vi "dual_color_2D_AFM_synched.vi"() -> ()   [LabVIEW 2017]
uses:
  <vilib>/DAQmx/write.llb/DAQmx Write (Analog DBL 1Chan 1Samp).vi
  <vilib>/DAQmx/write.llb/DAQmx Write (Analog 2D DBL NChan NSamp).vi
  <vilib>/DAQmx/write.llb/DAQmx Write (Analog 1D DBL NChan 1Samp).vi
  <vilib>/DAQmx/create/channels.llb/DAQmx Create Channel (AO-Voltage-Basic).vi
  <vilib>/DAQmx/miscellaneous.llb/DAQmx Fill In Error Info.vi
  <vilib>/DAQmx/configure/timing.llb/DAQmx Timing (Sample Clock).vi
  <vilib>/DAQmx/configure/trigger.llb/DAQmx Start Trigger (Digital Edge).vi
  <resource>/objmgr/daqmx.rc
panel:
  out "Focal Distance (um)":dbl
  out "Diopter":dbl
  in  "ETL3 (v) [4.76V allows light passing through unaltered]":dbl(slide)=4.76 min=-10.0 max=10.0 step=0.01 scale=-10.0..10.0
  in  "Y multiplier":dbl=1.0
  in  "X multiplier":dbl=-1.0
  in  "Y (v)":dbl(slide) min=-10.0 max=10.0 step=0.01 scale=-10.0..10.0
  in  "X (v)":dbl(slide) min=-10.0 max=10.0 step=0.01 scale=-10.0..10.0
  in  "Combined Movement (v)\nEquation: X * X Multiplier + Y * Y Multiplier":dbl(slide) min=-10.0 max=10.0 step=0.01 scale=-10.0..10.0
  out "Expected AFM Frequency (HZ)":dbl
  in  "Listbox 2":i32(listbox)=3
  in  "Listbox":i32(listbox)=1
  in  "Laser 2 (0-10v)":dbl=3.0
  in  "Laser 1 (0-10v)":dbl=3.0
  in  "OFF Time(ms)":dbl=100.0
  in  "ON Time(ms)":dbl=300.0
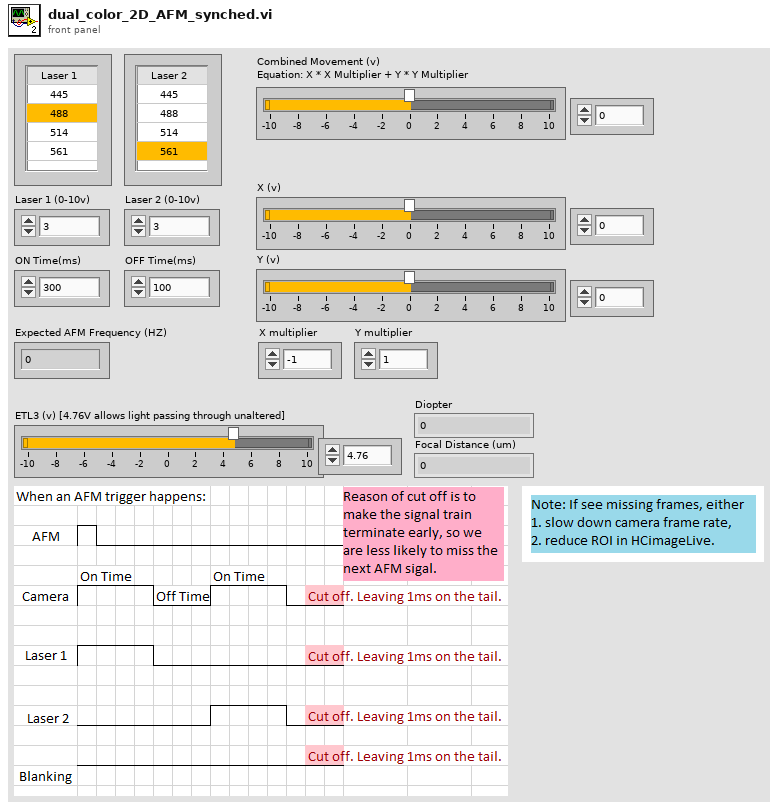
[diagram p1: front panel]
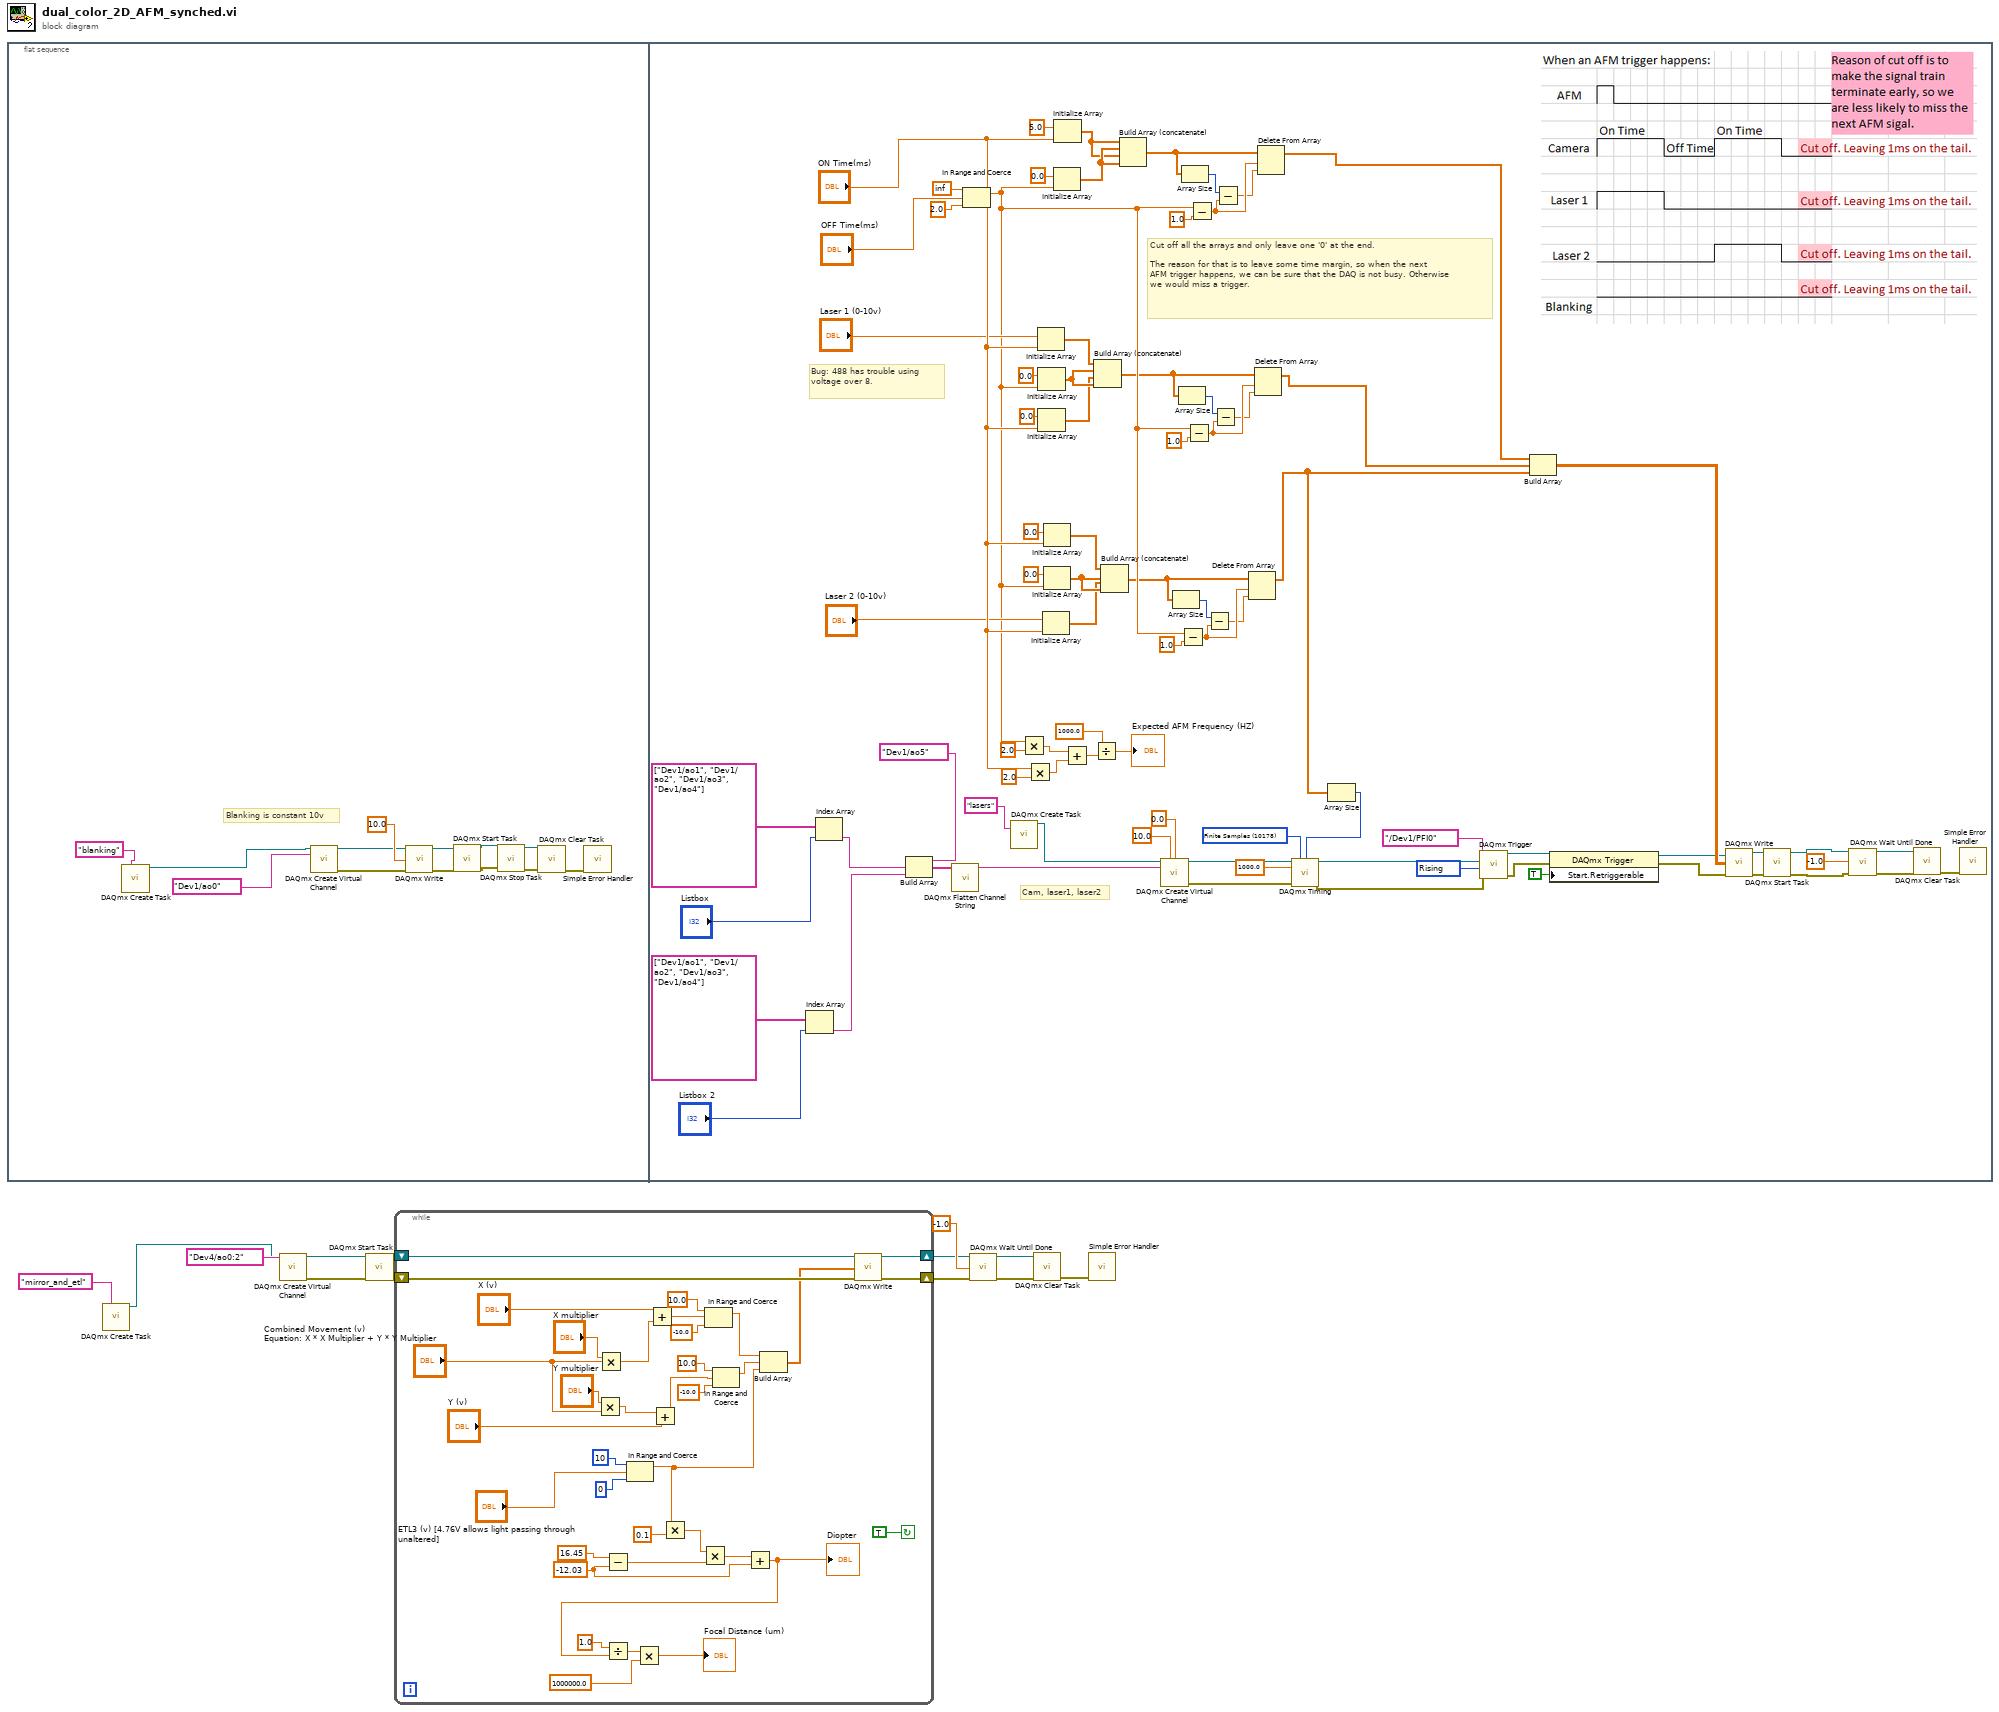
[diagram p0: block diagram]
diagram:
  n1 = flat-sequence {
    frame #0 {
      # "Blanking is constant 10v"
      n2 = call <vilib>:"DAQmx Create Task.vi"("new task name"="blanking" ("name to assign")) -> ("task out"=w16:refnum<k21>)  [unwired: 13 in, 1 out]
      n3 = call-poly <vilib>:"DAQmx Create Virtual Channel.vi"("task in"=w16, "physical channels"=tag "Dev1/ao0") -> ("task out"=w24:refnum<k21>, "error out"=w23:errorcluster)  [unwired: 12 in]
      n4 = call-poly <vilib>:"DAQmx Write.vi"("task/channels in"=w24, "data"=10.0, "error in"=w23) -> ("task out"=w22:refnum<k21>, "error out"=w21:errorcluster)  [unwired: 10 in, 1 out]
      n5 = call <vilib>:"DAQmx Start Task.vi"("task/channels in"=w22, "error in"=w21) -> ("task out"=w15:refnum<k21>, "error out"=w14:errorcluster)  [unwired: 12 in]
      n6 = call <vilib>:"DAQmx Stop Task.vi"("task/channels in"=w15, "error in"=w14) -> ("task out"=w20:refnum<k21>, "error out"=w19:errorcluster)  [unwired: 12 in]
      n7 = call <vilib>:"DAQmx Clear Task.vi"("task in"=w20, "error in"=w19) -> ("error out"=w26:errorcluster)  [unwired: 13 in]
      n8 = call <vilib>:"Simple Error Handler.vi"("error in (no error)"=w26) -> ()  [unwired: 4 in, 5 out]
    }
    frame #1 {
      w43 = 10280 items=["Rising"=10280, "Falling"=10171] ("edge")
      w39 = 10178 items=["Finite Samples"=10178, "Continuous Samples"=10123, "Hardware Timed Single Point"=12522] ("sample mode")
      # "Bug: 488 has trouble using voltage over 8."
      # "Cut off all the arrays and only leave one '0' at the end.\n\nThe reason for that is to leave some time margin, so when the next \nAFM trigger happens, we can be sure that the DAQ is not busy. Otherwise\nwe would miss a trigger."
      # "Cam, laser1, laser2"
      n9 = Index Array(array=tag[] ["Dev1/ao1", "Dev1/ao2", "Dev1/ao3", "Dev1/ao4"], index="Listbox 2") -> (element=w102:tag)
      n10 = Index Array(array=tag[] ["Dev1/ao1", "Dev1/ao2", "Dev1/ao3", "Dev1/ao4"], index="Listbox") -> (element=w101:tag)
      n11 = Build Array(tag "Dev1/ao5" ("physical channels"), w101, w102) -> (w103:tag[])
      n12 = call <vilib>:"DAQmx Flatten Channel String.vi"("names in"=w103) -> ("names out"=w106:string)  [unwired: 13 in, 1 out]
      n13 = In Range and Coerce(upper limit=inf, x="OFF Time(ms)", lower limit=2.0) -> (coerced(x)=w88:dbl)  [unwired: 1 out]
      n14 = call <vilib>:"DAQmx Create Task.vi"("new task name"="lasers" ("name to assign")) -> ("task out"=w108:refnum<k21>)  [unwired: 13 in, 1 out]
      n15 = Multiply(x=w88, y=2.0) -> (x*y=w90:dbl)
      n16 = Multiply(x="ON Time(ms)", y=2.0) -> (x*y=w89:dbl)
      n17 = Initialize Array("Laser 1 (0-10v)", "ON Time(ms)") -> (w59:dbl[])
      n18 = Initialize Array(0.0 ("element"), w88) -> (w61:dbl[])
      n19 = Initialize Array(0.0 ("element"), "ON Time(ms)") -> (w60:dbl[])
      n20 = Initialize Array("Laser 2 (0-10v)", "ON Time(ms)") -> (w67:dbl[])
      n21 = Initialize Array(0.0 ("element"), "ON Time(ms)") -> (w66:dbl[])
      n22 = Initialize Array(0.0 ("element"), w88) -> (w68:dbl[])
      n23 = Initialize Array(0.0 ("element"), w88) -> (w54:dbl[])
      n24 = Initialize Array(5.0 ("element"), "ON Time(ms)") -> (w53:dbl[])
      n25 = Add(x=w90, y=w89) -> (x+y=w91:dbl)
      n26 = Divide(x=1000.0, y=w91) -> (x/y=→"Expected AFM Frequency (HZ)":dbl)
      n27 = Build Array (concatenate)(w59, w61, w60, w61) -> (w65:dbl[])
      n28 = Build Array (concatenate)(w66, w68, w67, w68) -> (w72:dbl[])
      n29 = Build Array (concatenate)(w53, w54, w53, w54) -> (w55:dbl[])
      n30 = call-poly <vilib>:"DAQmx Create Virtual Channel.vi"("task in"=w108, "maximum value"=10.0, "minimum value"=0.0, "physical channels"=w106) -> ("task out"=w80:refnum<k21>, "error out"=w81:errorcluster)  [unwired: 10 in]
      n31 = Array Size(array=w72) -> (size(s)=w69:i32)
      n32 = Array Size(array=w65) -> (size(s)=w62:i32)
      n33 = Subtract(x=w88, y=1.0) -> (x-y=w71:dbl)
      n34 = Array Size(array=w55) -> (size(s)=w56:i32)
      n35 = Subtract(x=w88, y=1.0) -> (x-y=w64:dbl)
      n36 = Subtract(x=w88, y=1.0) -> (x-y=w58:dbl)
      n37 = Subtract(x=w69, y=w71) -> (x-y=w70:dbl)
      n38 = Subtract(x=w62, y=w64) -> (x-y=w63:dbl)
      n39 = Subtract(x=w56, y=w58) -> (x-y=w57:dbl)
      n40 = Delete From Array(array=w72, length=w71, index=w70) -> (array with subset deleted=w95:dbl[])  [unwired: 1 out]
      n41 = Delete From Array(array=w65, length=w64, index=w63) -> (array with subset deleted=w93:dbl[])  [unwired: 1 out]
      n42 = Delete From Array(array=w55, length=w58, index=w57) -> (array with subset deleted=w92:dbl[])  [unwired: 1 out]
      n43 = Array Size(array=w95) -> (size(s)=w107:i32)
      n44 = call-poly <vilib>:"DAQmx Timing.vi"("task/channels in"=w80, "sample mode"=w39, "samples per channel"=w107, "rate"=1000.0, "error in"=w81) -> ("task out"=w82:refnum<k21>, "error out"=w83:errorcluster)  [unwired: 9 in]
      n45 = call-poly <vilib>:"DAQmx Trigger.vi"("task/channels in"=w82, "source"=tag "/Dev1/PFI0", "edge"=w43, "error in"=w83) -> ("task out"=w84:refnum<k21>, "error out"=w87:errorcluster)  [unwired: 10 in]
      n46 = Build Array(w92, w93, w95) -> (w94:dbl[][])
      n47 = property class="DAQmx Trigger"(reference=w84, error in=w87, "Start.Retriggerable"=TRUE) -> (reference out=w85:refnum<k21>, error out=w86:errorcluster)
      n48 = call-poly <vilib>:"DAQmx Write.vi"("task/channels in"=w85, "data"=w94, "error in"=w86) -> ("task out"=w78:refnum<k21>, "error out"=w79:errorcluster)  [unwired: 10 in, 1 out]
      n49 = call <vilib>:"DAQmx Start Task.vi"("task/channels in"=w78, "error in"=w79) -> ("task out"=w77:refnum<k21>, "error out"=w76:errorcluster)  [unwired: 12 in]
      n50 = call <vilib>:"DAQmx Wait Until Done.vi"("task/channels in"=w77, "timeout (sec)"=-1.0, "error in"=w76) -> ("task out"=w74:refnum<k21>, "error out"=w75:errorcluster)  [unwired: 11 in]
      n51 = call <vilib>:"DAQmx Clear Task.vi"("task in"=w74, "error in"=w75) -> ("error out"=w73:errorcluster)  [unwired: 13 in]
      n52 = call <vilib>:"Simple Error Handler.vi"("error in (no error)"=w73) -> ()  [unwired: 4 in, 5 out]
    }
  }
  n53 = call <vilib>:"DAQmx Create Task.vi"("new task name"="mirror_and_etl" ("name to assign")) -> ("task out"=w1:refnum<k21>)  [unwired: 13 in, 1 out]
  n54 = call-poly <vilib>:"DAQmx Create Virtual Channel.vi"("task in"=w1, "physical channels"=tag "Dev4/ao0:2") -> ("task out"=w6:refnum<k21>, "error out"=w5:errorcluster)  [unwired: 12 in]
  n55 = call <vilib>:"DAQmx Start Task.vi"("task/channels in"=w6, "error in"=w5) -> ("task out"=w8:refnum<k21>, "error out"=w7:errorcluster)  [unwired: 12 in]
  n56 = while {
    shift-right: [w142] -> w3
    shift-left: w8 -> [w144]
    shift-right: [w141] -> w4
    shift-left: w7 -> [w143]
    stop <- TRUE continue-if-true
    w118 = -12.03 ("x")
    n57 = Multiply(x="Y multiplier", y="Combined Movement (v)\nEquation: X * X Multiplier + Y * Y Multiplier") -> (x*y=w129:dbl)
    n58 = Multiply(x="X multiplier", y="Combined Movement (v)\nEquation: X * X Multiplier + Y * Y Multiplier") -> (x*y=w138:dbl)
    n59 = Subtract(x=16.45 ("y"), y=w118) -> (x-y=w120:dbl)
    n60 = In Range and Coerce(upper limit=10, x="ETL3 (v) [4.76V allows light passing through unaltered]", lower limit=0) -> (coerced(x)=w117:dbl)  [unwired: 1 out]
    n61 = Add(x="X (v)", y=w138) -> (x+y=w137:dbl)
    n62 = Add(x=w129, y="Y (v)") -> (x+y=w131:dbl)
    n63 = Multiply(x=w117, y=0.1) -> (x*y=w121:dbl)
    n64 = Multiply(x=w121, y=w120) -> (x*y=w119:dbl)
    n65 = In Range and Coerce(upper limit=10.0, x=w137, lower limit=-10.0) -> (coerced(x)=w134:dbl)  [unwired: 1 out]
    n66 = In Range and Coerce(upper limit=10.0, x=w131, lower limit=-10.0) -> (coerced(x)=w130:dbl)  [unwired: 1 out]
    n67 = Add(x=w119, y=w118) -> (x+y=w112:dbl)
    "Diopter" <- w112
    n68 = Divide(x=1.0, y=w112) -> (x/y=w127:dbl)
    n69 = Multiply(x=w127, y=1000000.0) -> (x*y=→"Focal Distance (um)":dbl)
    n70 = Build Array(w134, w130, w117) -> (w140:dbl[])
    n71 = call-poly <vilib>:"DAQmx Write.vi"("task/channels in"=w144, "data"=w140, "error in"=w143) -> ("task out"=w142:refnum<k21>, "error out"=w141:errorcluster)  [unwired: 10 in, 1 out]
  }
  n72 = call <vilib>:"DAQmx Wait Until Done.vi"("task/channels in"=w3, "timeout (sec)"=-1.0, "error in"=w4) -> ("task out"=w12:refnum<k21>, "error out"=w11:errorcluster)  [unwired: 11 in]
  n73 = call <vilib>:"DAQmx Clear Task.vi"("task in"=w12, "error in"=w11) -> ("error out"=w13:errorcluster)  [unwired: 13 in]
  n74 = call <vilib>:"Simple Error Handler.vi"("error in (no error)"=w13) -> ()  [unwired: 4 in, 5 out]
